vi "CalculateGap.vi"(9 "feature":T1, 10 "channel":T3, 11 "waveform data":waveform(sgl)) -> (2 "gap":dbl)   [LabVIEW 2017, in "AnalysisHelper.lvlib"]
uses:
  <vilib>/addons/InsightCM/Utilities/Analysis/Shared/AnalysisHelper.lvlib
  <vilib>/addons/InsightCM/Utilities/Analysis/Shared/controls/Channel.ctl
  <vilib>/addons/InsightCM/Utilities/Analysis/Shared/controls/SpeedType.ctl
  <vilib>/addons/InsightCM/Utilities/Analysis/Shared/controls/Feature.ctl
  <vilib>/addons/InsightCM/Utilities/Analysis/Shared/controls/AmplitudeScale.ctl
  <vilib>/addons/InsightCM/Utilities/Analysis/Vibration/VibrationAnalysisFunctions.lvlib
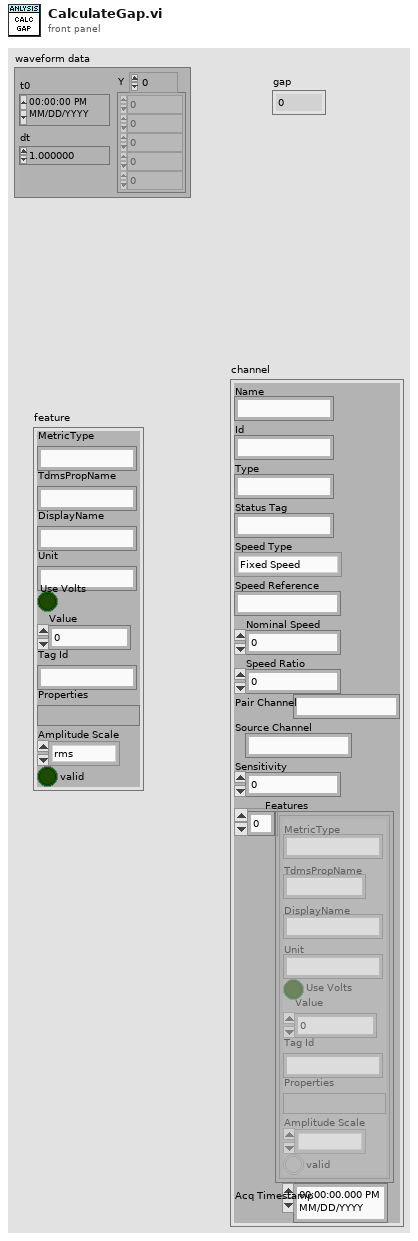
[diagram p1: front panel]
types:
  T1 = typedef "AnalysisHelper.lvlib/Feature.ctl" = cluster{"MetricType":string, "TdmsPropName":string, "DisplayName":string, "Unit":string, "Use Volts":bool, "Value":dbl, "Tag Id":string, "Properties":variant, "Amplitude Scale":T2, "valid":bool}
  T2 = typedef "AnalysisHelper.lvlib/AmplitudeScale.ctl" = enum16{"rms", "peak", "pk-pk"}
  T3 = typedef "AnalysisHelper.lvlib/Channel.ctl" = cluster{"Name":string, "Id":string, "Type":string, "Status Tag":string, "Speed Type":T4, "Speed Reference":string, "Nominal Speed":dbl, "Speed Ratio":dbl, "Pair Channel":string, "Source Channel":string, "Sensitivity":dbl, "Features":T1[], "Acq Timestamp":timestamp}
  T4 = typedef "AnalysisHelper.lvlib/SpeedType.ctl" = enum16{"Fixed Speed", "Tachometer"}
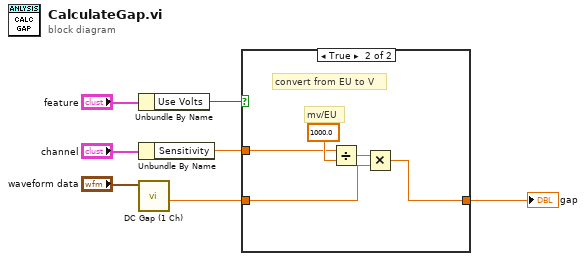
[diagram p0: block diagram]
diagram:
  n1 = Unbundle By Name("feature") -> ("Use Volts"=w1:bool)
  n2 = Unbundle By Name("channel") -> ("Sensitivity"=w3:dbl)
  n3 = call <vilib>:"DC Gap (1 Ch).vi"("Waveform"="waveform data") -> ("DC gap"=w5:sgl)  [unwired: 8 in, 2 out]
  n4 = case shown="True" w1 {
    tunnel: [w8 w13] -> w7
    tunnel: w3 -> [_ w9]
    tunnel: w5 -> [w8 w10]
    frame False {
    }
    frame True {
      # "convert from EU to V"
      # "mv/EU"
      n5 = Divide(x=w9, y=1000.0) -> (x/y=w11:dbl)
      n6 = Multiply(x=w11, y=w10) -> (x*y=w13:dbl)
    }
  }
  "gap" <- w7
